vi "Main.vi"   [LabVIEW 2021]
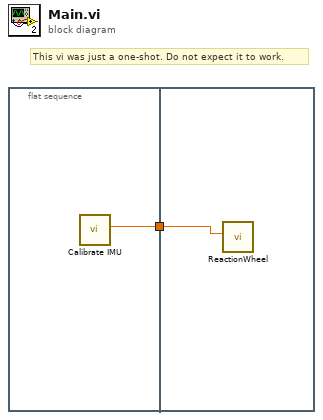
[diagram p0: block diagram]
diagram:
  # "This vi was just a one-shot. Do not expect it to work."
  n1 = flat-sequence {
    tunnel: [w2] -> w1
    tunnel: w1 -> [w3]
    frame #0 {
      n2 = call "Calibrate IMU.vi"() -> ("Roll bias (deg)"=w2:dbl)  [unwired: 11 in]
    }
    frame #1 {
      n3 = call "ReactionWheel.vi"("Roll bias (deg)"=w3) -> ()  [unwired: 11 in]
    }
  }
